vi "Force Outputs Mapping.vi"(8 "error in (no error)":errorcluster, 11 "Device Item Ref in":T1 format="%.0x") -> (0 "error out":errorcluster, 3 "Device Item Ref out":T1 format="%.0x")   [LabVIEW 2019, in "Control Addon Shared.lvlib"]
uses:
  Control Addon Shared.lvlib
  <vilib>/NI VeriStand/Custom Device API/Custom Device Item Ref.ctl
  Constants.vi
  <vilib>/NI/NI VeriStand Advanced SysDef API/_SubVIs/SysDef.Search.GUIDs.vi
  <vilib>/NI/NI VeriStand Advanced SysDef API/SysDef API/Advanced System Definition.lvlib
  <vilib>/NI VeriStand/Custom Device API/Custom Device API.lvlib
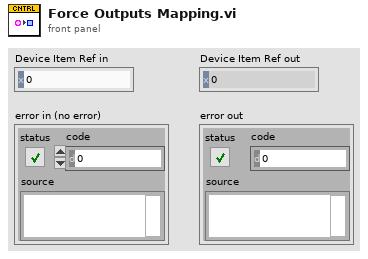
[diagram p1: front panel]
types:
  T1 = typedef "Custom Device API.lvlib/Custom Device Item Ref.ctl" = u64
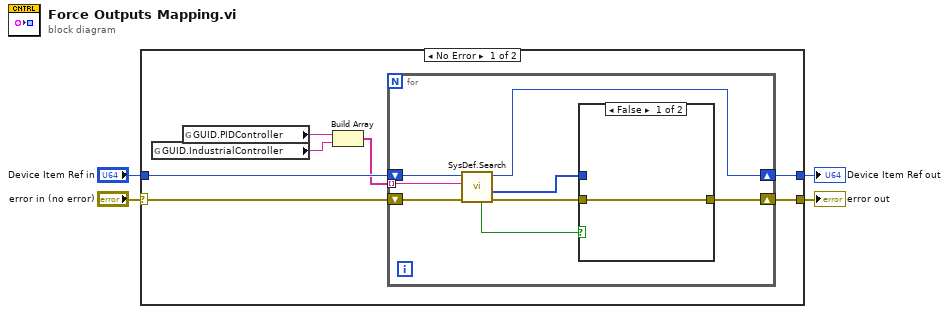
[diagram p0: block diagram]
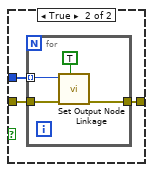
[diagram p2: hidden frame]
diagram:
  n1 = case shown="No Error" "error in (no error)" {
    selector: "error in (no error)" -> [w9 w29]
    tunnel: [w11 w29] -> w1
    tunnel: "Device Item Ref in" -> [w10 w28]
    tunnel: [w5 w28] -> w2
    frame No Error {
      n2 = global read "Constants.vi" "GUID.IndustrialController"() -> (w7:string)
      n3 = global read "Constants.vi" "GUID.PIDController"() -> (w8:string)
      n4 = Build Array(w8, w7) -> (w6:string[])
      n5 = for {
        tunnel: w6 -> [w16] mode=indexing
        shift-right: [w19] -> w11
        shift-left: w9 -> [w17]
        shift-right: [w12] -> w5
        shift-left: w10 -> [w18]
        n6 = call-poly <vilib>:"SysDef.Search.vi"("error in (no error)"=w17, "GUID"=w16, "nodeID"=w18) -> ("error out"=w14:errorcluster, "Values Out"=w15:u64[], "nodeID out"=w12:u64, "Found?"=w13:bool)  [unwired: 5 in]
        n7 = case shown="False" w13 {
          tunnel: [w20 w23] -> w19
          tunnel: w15 -> [_ w22]
          tunnel: w14 -> [w20 w21]
          frame False {
          }
          frame True {
            n8 = for {
              tunnel: [w26] -> w23
              tunnel: w22 -> [w25] mode=indexing
              tunnel: w21 -> [w24]
              n9 = call "Set Output Node Linkage.vi"("Add?"=TRUE, "error in"=w24, "Section Ref in"=w25) -> ("error out"=w26:errorcluster)  [unwired: 7 in, 1 out]
            }
          }
        }
      }
    }
    frame Error {
    }
  }
  "Device Item Ref out" <- w2
  "error out" <- w1
